vi "file_LabVIEW_2.vi"() -> ()   [LabVIEW 2022 SP3]
uses:
  <vilib>/Instr/_visa.llb/VISA Configure Serial Port (Instr).vi
panel:
  out "Grafik Encoder":i32(graph)
  out "read buffer":string
  in  "Slide":i16(slide) scale=-255.0..255.0
  in  "VISA resource name":refnum<visa-resource-name>
  in  "stop":bool
  out "Grafik PWM":i16(graph)
  # "KONTROL PWM & ENCODER"
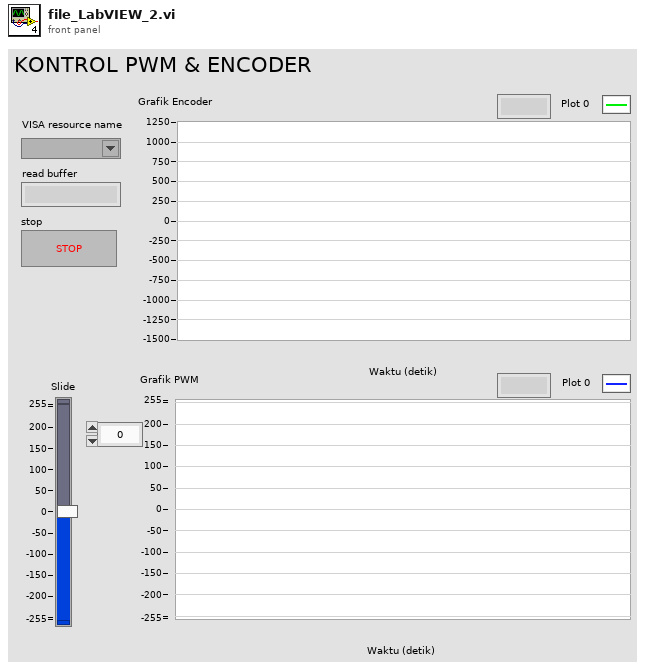
[diagram p1: front panel]
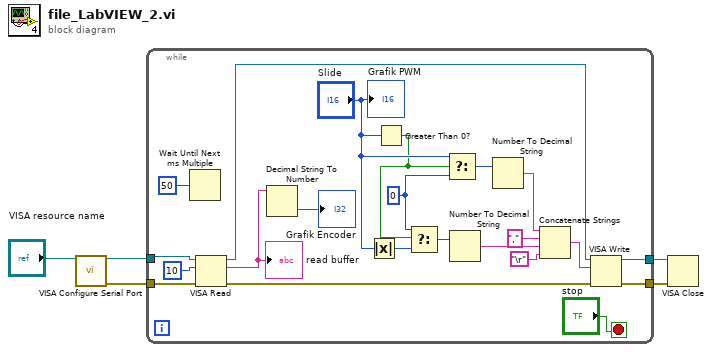
[diagram p0: block diagram]
diagram:
  n1 = call-poly "VISA Configure Serial Port"("VISA resource name"="VISA resource name") -> ("VISA resource name out"=w3:refnum<visa-resource-name>, "error out"=w2:errorcluster)  [unwired: 13 in]
  n2 = while {
    tunnel: [w27] -> w5
    tunnel: [w26] -> w4
    tunnel: w3 -> [w13]
    tunnel: w2 -> [w14]
    stop <- "stop" stop-if-true
    w25 = 0
    n3 = Wait Until Next ms Multiple(millisecond multiple=u32 50) -> ()  [unwired: 1 out]
    n4 = VISA Read(VISA resource name=w13, byte count=u32 10, error in (no error)=w14) -> (VISA resource name out=w11:refnum<visa-resource-name>, read buffer=w8:string, error out=w12:errorcluster)  [unwired: 1 out]
    "read buffer" <- w8
    n5 = Decimal String To Number(string=w8) -> (number=→"Grafik Encoder":i32)  [unwired: 2 in, 1 out]
    n6 = Absolute Value(x="Slide") -> (abs(x)=w24:i16)
    n7 = Greater Than 0?(x="Slide") -> (x > 0?=w7:bool)
    n8 = Select(t=w25, s=w7, f=w24) -> (s? t:f=w22:i32)
    n9 = Select(t="Slide", s=w7, f=w25) -> (s? t:f=w23:i32)
    n10 = Number To Decimal String(number=w22) -> (decimal integer string=w19:string)  [unwired: 1 in]
    n11 = Number To Decimal String(number=w23) -> (decimal integer string=w21:string)  [unwired: 1 in]
    n12 = Concatenate Strings "Concatenate Strings"(w21, "," ("string"), w19, "\r") -> (w18:string)
    n13 = VISA Write(VISA resource name=w11, write buffer=w18, error in (no error)=w12) -> (VISA resource name out=w26:refnum<visa-resource-name>, error out=w27:errorcluster)  [unwired: 1 out]
    "Grafik PWM" <- "Slide"
  }
  n14 = VISA Close(VISA resource name=w4, error in (no error)=w5) -> ()  [unwired: 1 out]
